vi "Specs.vi"(9 "Select Spec":string(combo), 10 "body":string, 11 "ComboBox in":refnum<vi>) -> (1 "Value":string, 2 "Label":string, 3 "Unit":string, 4 "Created":dbl, 5 "ID":string, 6 "Model":string)   [LabVIEW 2019]
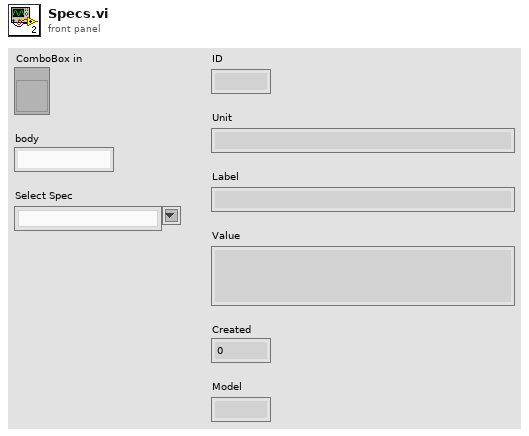
[diagram p1: front panel]
types:
  T1 = cluster{"specs":cluster{"unit":string, "id":string, "label":string, "value":string}[], "id":string, "model":string, "created":i32}
  T2 = cluster{"unit":string, "id":string, "label":string, "value":string}[]
  T3 = cluster{"unit":string, "id":string, "label":string, "value":string}
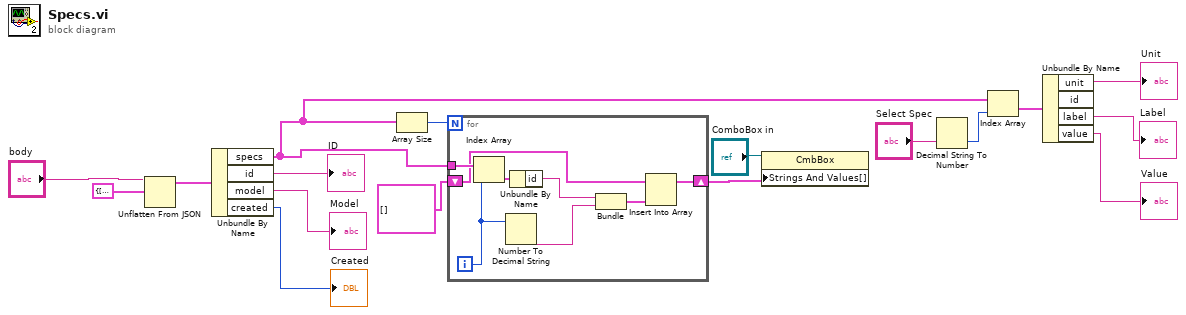
[diagram p0: block diagram]
diagram:
  n1 = Unflatten From JSON(JSON string="body", type and defaults=T1 {"specs"=[], "id"="", "model"="", "created"=0}) -> (value=w4:T1)  [unwired: 5 in, 1 out]
  n2 = Unbundle By Name(w4) -> ("specs"=w13:T2, "id"=→"ID":string, "model"=→"Model":string, "created"=→"Created":i32)
  n3 = Array Size(array=w13) -> (size(s)=w8:i32)
  n4 = for {
    N: w8 -> [_]
    tunnel: w13 -> [w25]
    shift-right: [w20] -> w9
    shift-left: cluster{"id":string, string}[] [] -> [w21]
    i -> [w19]
    n5 = Index Array(array=w25, index=w19) -> (element=w24:T3)
    n6 = Number To Decimal String(number=w19) -> (decimal integer string=w18:string)  [unwired: 1 in]
    n7 = Unbundle By Name(w24) -> ("id"=w23:string)
    n8 = Bundle("id"=w23, w18) -> (w22:cluster{"id":string, string})  [unwired: 1 in]
    n9 = Insert Into Array(array=w21, new element=w22) -> (w20:cluster{"id":string, string}[])  [unwired: 1 in]
  }
  n10 = property on="Property Node" class="CmbBox"(reference="ComboBox in", "Strings And Values[]"=w9) -> ()  [unwired: 1 in, 2 out]
  n11 = Decimal String To Number(string="Select Spec") -> (number=w12:i32)  [unwired: 2 in, 1 out]
  n12 = Index Array(array=w13, index=w12) -> (element=w14:T3)
  n13 = Unbundle By Name(w14) -> ("unit"=→"Unit":string, "label"=→"Label":string, "value"=→"Value":string)  [unwired: 1 out]
